vi "formulanodes.vi"() -> ()   [LabVIEW 2015]
panel:
  in  "stop":bool
  out "Numeric Indicator 2":dbl
  out "Numeric Indicator":dbl
  out "String 2":string
  out "String":string
  in  "X2":dbl
  in  "Y2":dbl
  in  "Y1":dbl
  in  "X1":dbl
  out "XY Graph":cluster{i32[], dbl[]}(graph)
  # "x +"
  # "Y ="
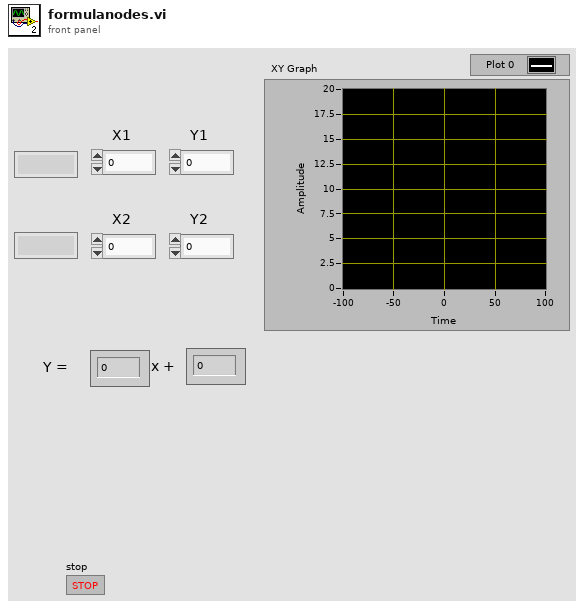
[diagram p1: front panel]
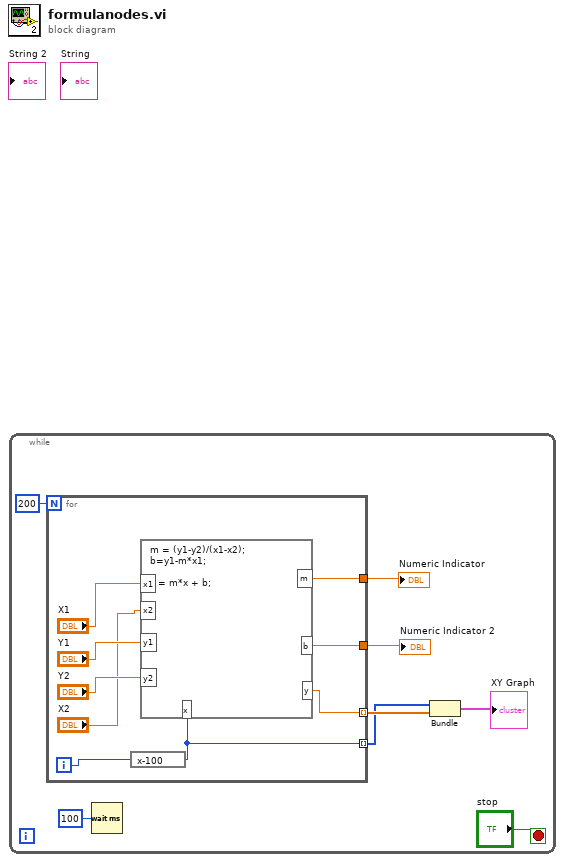
[diagram p0: block diagram]
diagram:
  n1 = while {
    stop <- "stop" stop-if-true
    n2 = for {
      N: 200 -> [_]
      tunnel: [w17] -> w6
      tunnel: [w16] -> w5
      tunnel: [w14] -> w2 mode=indexing
      tunnel: [w13] -> w3 mode=indexing
      i -> [w15]
      n3 = expression code="x-100"(w15) -> (w14:i32)
      n4 = formula code="m = (y1-y2)/(x1-x2);\nb=y1-m*x1;\n\ny = m*x + b;"("x1"="X1", "x2"="X2", "y1"="Y1", "y2"="Y2", "x"=w14) -> ("m"=w17:dbl, "b"=w16:dbl, "y"=w13:dbl)
    }
    "Numeric Indicator" <- w6
    "Numeric Indicator 2" <- w5
    n5 = Wait (ms)(milliseconds to wait=u32 100) -> ()  [unwired: 1 out]
    n6 = Bundle(w2, w3) -> (→"XY Graph":cluster{i32[], dbl[]})  [unwired: 1 in]
  }
